vi "AM Pump Control.vi"(7 "input cluster":T1, 8 "error in (no error)":errorcluster, 11 "Times":dbl[](array[numeric])) -> (0 "error out":errorcluster)   [LabVIEW 2020]
uses:
  support/Message Queue/All Message Queues.ctl
  support/Message Queue/Message Cluster.ctl
  support/Message Queue/Message Queue.lvlib
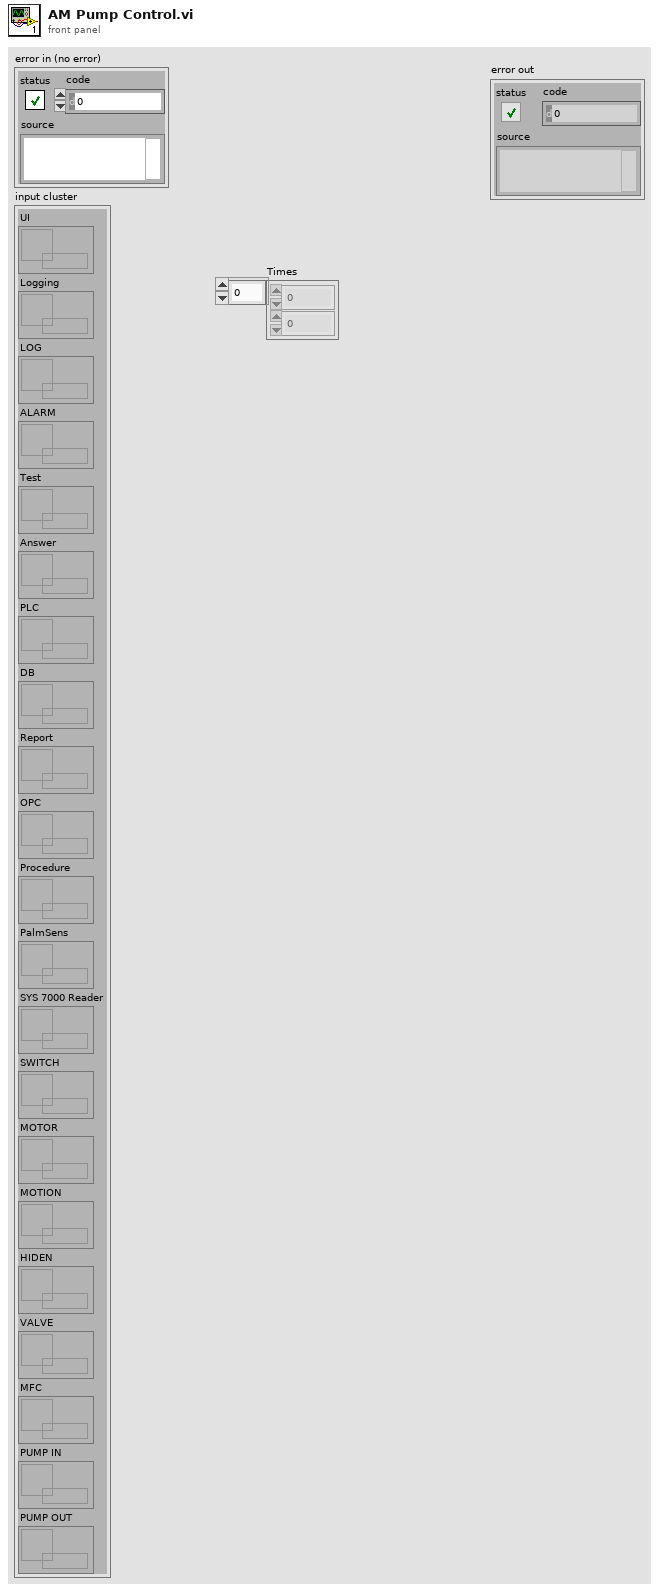
[diagram p1: front panel]
types:
  T1 = typedef "Message Queue.lvlib/All Message Queues.ctl" = cluster{"UI":refnum<queue>, "Logging":refnum<queue>, "LOG":refnum<queue>, "ALARM":refnum<queue>, "Test":refnum<queue>, "Answer":refnum<queue>, "PLC":refnum<queue>, "DB":refnum<queue>, "Report":refnum<queue>, "OPC":refnum<queue>, "Procedure":refnum<queue>, "PalmSens":refnum<queue>, "SYS 7000 Reader":refnum<queue>, "SWITCH":refnum<queue>, "MOTOR":refnum<queue>, "MOTION":refnum<queue>, "HIDEN":refnum<queue>, "VALVE":refnum<queue>, "MFC":refnum<queue>, "PUMP IN":refnum<queue>, "PUMP OUT":refnum<queue>}
  T2 = cluster{"Type CMD":string, "Mode CMD":string, "Main CMD":string}
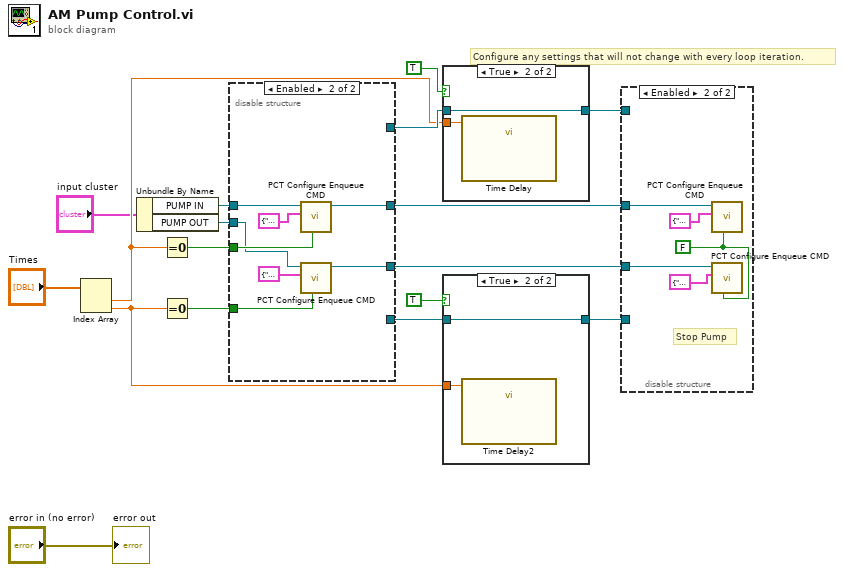
[diagram p0: block diagram]
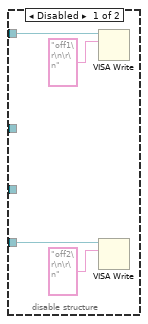
[diagram p2: hidden frame]
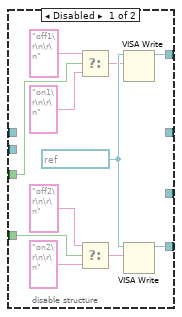
[diagram p3: hidden frame]
diagram:
  # "Configure any settings that will not change with every loop iteration."
  n1 = Index Array(array="Times") -> (element #1=w10:dbl, element #2=w9:dbl)  [unwired: 2 in]
  n2 = Unbundle By Name("input cluster") -> ("PUMP IN"=w4:refnum<queue>, "PUMP OUT"=w3:refnum<queue>)
  n3 = Equal To 0?(x=w10) -> (x = 0?=w6:bool)
  n4 = Equal To 0?(x=w9) -> (x = 0?=w8:bool)
  n5 = disable-structure shown="Enabled" {
    disable-tunnel: [w28 _] -> w15
    disable-tunnel: [w26 _] -> w14
    disable-tunnel: w8 -> [w22 w33]
    disable-tunnel: w6 -> [w18 w34]
    disable-tunnel: w4 -> [_ w32]
    disable-tunnel: w3 -> [_ w31]
    disable-tunnel: [_ w30] -> w2
    disable-tunnel: [_ w29] -> w1
    frame Disabled {
      w27 = refnum<visa-resource-name> "COM14" ("VISA resource")
      n6 = Select(t="off1\r\n\r\n" ("concatenated string"), s=w18, f="on1\r\n\r\n" ("concatenated string")) -> (s? t:f=w23:string)
      n7 = Select(t="off2\r\n\r\n" ("concatenated string"), s=w22, f="on2\r\n\r\n" ("concatenated string")) -> (s? t:f=w19:string)
      n8 = VISA Write(VISA resource name=w27, write buffer=w23) -> (VISA resource name out=w28:refnum<visa-resource-name>)  [unwired: 1 in, 2 out]
      n9 = VISA Write(VISA resource name=w27, write buffer=w19) -> (VISA resource name out=w26:refnum<visa-resource-name>)  [unwired: 1 in, 2 out]
    }
    frame Enabled {
      n10 = call "PCT Configure Enqueue CMD.vi"("Parameter Data"=w34, "CMD"=T2 {"Type CMD"="Run", "Mode CMD"="", "Main CMD"="Action-Status"}, "CMD Queue in"=w32) -> ("CMD Queue out"=w30:refnum<queue>)  [unwired: 6 in, 2 out]
      n11 = call "PCT Configure Enqueue CMD.vi"("Parameter Data"=w33, "CMD"=T2 {"Type CMD"="Run", "Mode CMD"="", "Main CMD"="Action-Status"}, "CMD Queue in"=w31) -> ("CMD Queue out"=w29:refnum<queue>)  [unwired: 6 in, 2 out]
    }
  }
  n12 = case shown="True" TRUE {
    tunnel: w15 -> [w37 w39]
    tunnel: [w37 w39] -> w12
    tunnel: w10 -> [_ w38]
    frame False {
    }
    frame True {
      n13 = call "Time Delay"("Delay Time (s)"=w38) -> ()  [unwired: 10 in, 1 out]
    }
  }
  n14 = case shown="True" TRUE {
    tunnel: w14 -> [w40 w42]
    tunnel: [w40 w42] -> w13
    tunnel: w9 -> [_ w41]
    frame False {
    }
    frame True {
      n15 = call "Time Delay2"("Delay Time (s)"=w41) -> ()  [unwired: 10 in, 1 out]
    }
  }
  n16 = disable-structure shown="Enabled" {
    disable-tunnel: w13 -> [w45 _]
    disable-tunnel: w12 -> [w43 _]
    disable-tunnel: w2 -> [_ w48]
    disable-tunnel: w1 -> [_ w47]
    frame Disabled {
      n17 = VISA Write(VISA resource name=w43, write buffer="off1\r\n\r\n" ("concatenated string")) -> ()  [unwired: 1 in, 3 out]
      n18 = VISA Write(VISA resource name=w45, write buffer="off2\r\n\r\n" ("concatenated string")) -> ()  [unwired: 1 in, 3 out]
    }
    frame Enabled {
      w50 = FALSE
      # "Stop Pump"
      n19 = call "PCT Configure Enqueue CMD.vi"("Parameter Data"=w50, "CMD"=T2 {"Type CMD"="Run", "Mode CMD"="", "Main CMD"="Action-Status"}, "CMD Queue in"=w48) -> ()  [unwired: 6 in, 3 out]
      n20 = call "PCT Configure Enqueue CMD.vi"("Parameter Data"=w50, "CMD"=T2 {"Type CMD"="Run", "Mode CMD"="", "Main CMD"="Action-Status"}, "CMD Queue in"=w47) -> ()  [unwired: 6 in, 3 out]
    }
  }
  "error out" <- "error in (no error)"
